vi "Get Feature Names.vi"(8 "error in (no error)":errorcluster caption="entrée d'erreur (pas d'erreur)", 9 "doc":string, 10 "raw_documents":string[][](array[string]), 11 "CountVectorizer.lvclass":refnum<class "CountVectorizer.lvclass">) -> (0 "error out":errorcluster caption="sortie d'erreur", 2 "Data":T1, 3 "CountVectorizer.lvclass":refnum<class "CountVectorizer.lvclass">)   [LabVIEW 2020, in "CountVectorizer.lvclass"]
doc: "Array mapping from feature integer indices to feature name.\n\nReturns : \n\n- feature_names : list\nA list of feature names."
uses:
  CountVectorizer.lvclass
  CountVectorizer.lvclass/CountVectorizer.ctl
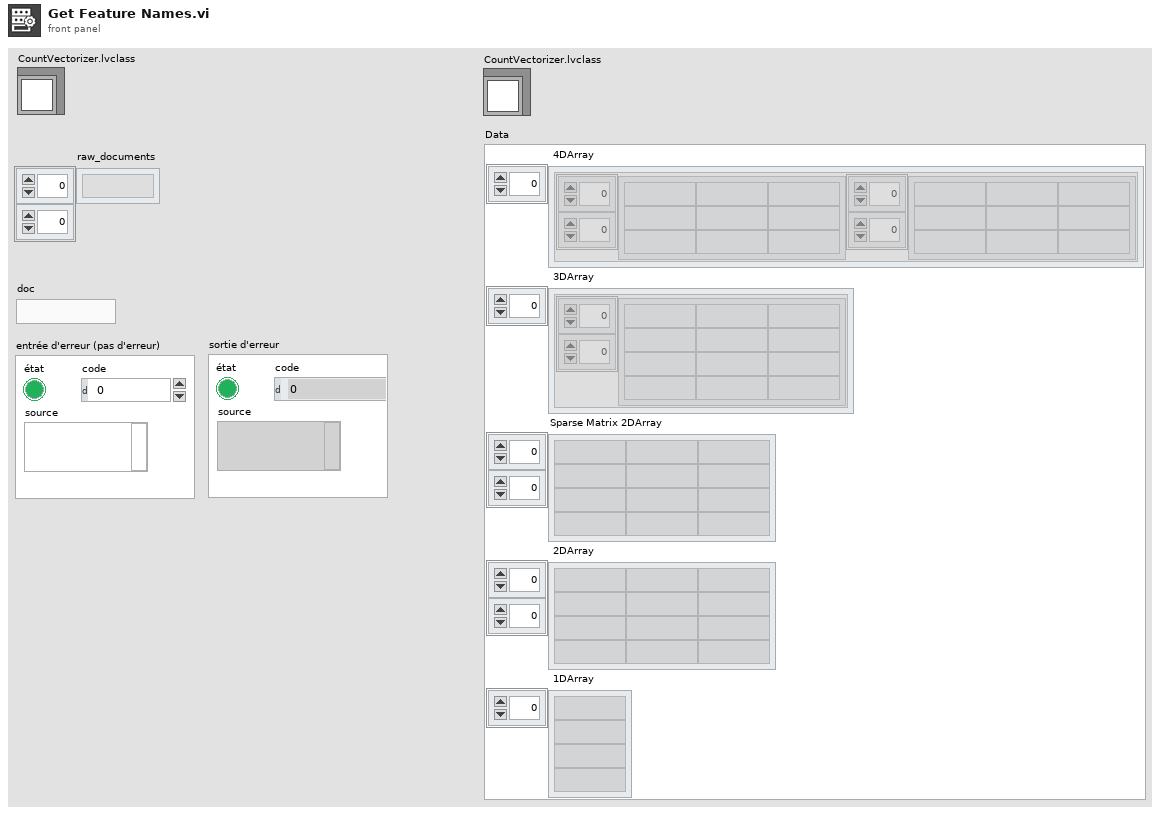
[diagram p1: front panel]
types:
  T1 = cluster{" 4DArray":cluster{"1":string[][], "2":string[][]}[], " 3DArray":cluster{"Tableau":string[][]}[], "Sparse Matrix 2DArray":string[][], " 2DArray":string[][], " 1DArray":string[]}
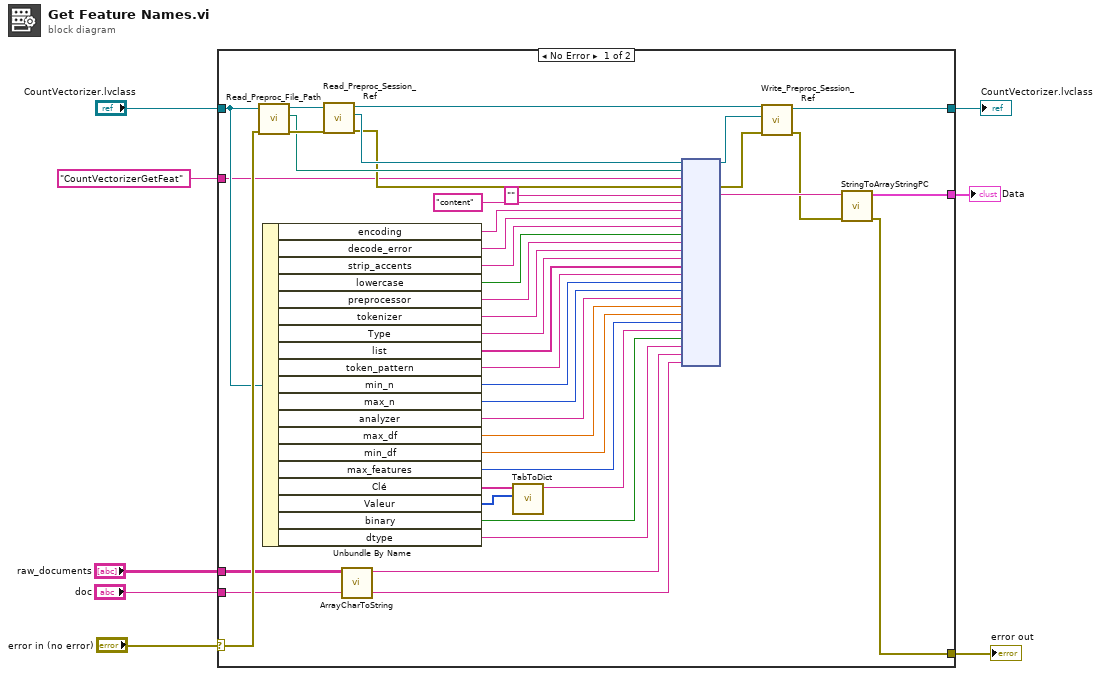
[diagram p0: block diagram]
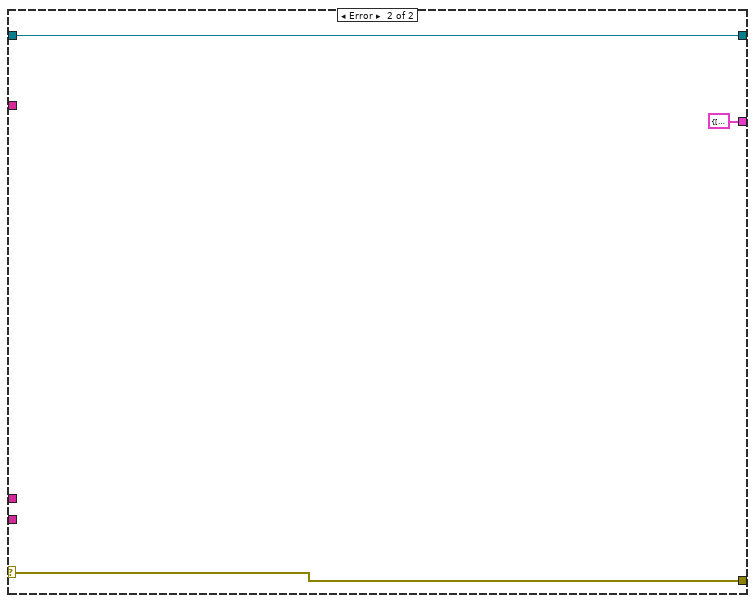
[diagram p2: hidden frame]
diagram:
  n1 = case shown="No Error" "error in (no error)" {
    selector: "error in (no error)" -> [w38 w52]
    tunnel: [w10 w52] -> w7
    tunnel: [w9 w51] -> w5
    tunnel: "CountVectorizer.lvclass" -> [w37 w51]
    tunnel: "CountVectorizerGetFeat" ("Fonction") -> [w36 _]
    tunnel: [w12 T1 {" 4DArray"=[], " 3DArray"=[], "Sparse Matrix 2DArray"=[], " 2DArray"=[], " 1DArray"=[]} ("Data")] -> w1
    tunnel: "raw_documents" -> [w15 _]
    tunnel: "doc" -> [w16 _]
    frame No Error {
      n2 = call-dynamic "Read_Preproc_File_Path.vi"("error in (no error)"=w38, "Python in"=w37) -> ("error out"=w48:errorcluster, "File_Path"=w47:path, "Python out"=w49:refnum<class "CountVectorizer.lvclass">)  [unwired: 7 in]
      n3 = Unbundle By Name(w37) -> ("encoding"=w40:string, "decode_error"=w39:string, "strip_accents"=w35:string, "lowercase"=w34:bool, "preprocessor"=w33:string, "tokenizer"=w32:string, "Type"=w31:string, "list"=w27:string[], "token_pattern"=w26:string, "min_n"=w25:i32, "max_n"=w24:i32, "analyzer"=w23:string, "max_df"=w22:dbl, "min_df"=w21:dbl, "max_features"=w20:i32, "Clé"=w29:string[], "Valeur"=w28:i32[], "binary"=w18:bool, "dtype"=w17:string)
      n4 = call-dynamic "Read_Preproc_Session_Ref.vi"("error in (no error)"=w48, "Python in"=w49) -> ("error out"=w45:errorcluster, "Session_ref"=w46:refnum<k35>, "Python out"=w44:refnum<class "CountVectorizer.lvclass">)  [unwired: 7 in]
      n5 = call "ArrayCharToString.vi"("TAB"=w15) -> ("Instruction"=w14:string)  [unwired: 10 in]
      n6 = call "TabToDict.vi"("Int Value"=w28, "String key"=w29) -> ("Dict with int value"=w19:string)  [unwired: 8 in, 1 out]
      n7 = node(w46, w47, w36, w45, "", "content", w40, w39, w35, w34, w33, w32, w31, w27, w26, w25, w24, w23, w22, w21, w20, w19, w18, w17, w14, w16) -> (w42:refnum<k35>, w43:errorcluster, w13:string)  [unwired: 21 in, 2 out]
      n8 = call-dynamic "Write_Preproc_Session_Ref.vi"("error in (no error)"=w43, "Session_ref"=w42, "Python in"=w44) -> ("error out"=w11:errorcluster, "Python out"=w9:refnum<class "CountVectorizer.lvclass">)  [unwired: 7 in]
      n9 = call "StringToArrayStringPC.vi"("sortie d'erreur"=w11, "Return value"=w13) -> ("sortie d'erreur"=w10:errorcluster, "Data"=w12:T1)  [unwired: 8 in]
    }
    frame Error {
    }
  }
  "error out" <- w7
  "CountVectorizer.lvclass" <- w5
  "Data" <- w1
